vi "Add.vi"(8 "error in (no error)":errorcluster, 9 "parent tag":string, 10 "Destinations in":refnum<class "IB_Destination.lvclass">[](array[class]), 11 "userFolder in":refnum<class "userFolder.lvclass">) -> (0 "error out":errorcluster, 1 "duplicate?":bool, 2 "Destinations out":refnum<class "IB_Destination.lvclass">[](array[class]), 3 "userFolder out":refnum<class "userFolder.lvclass">)   [LabVIEW 2020, in "userFolder.lvclass"]
uses:
  <vilib>/AppBuilder/IB_Classes/Destination/userFolder/userFolder.lvclass
  <vilib>/AppBuilder/IB_Classes/Destination/userFolder/userFolder.lvclass/userFolder.ctl
  <vilib>/AppBuilder/IB_Classes/Destination/IB_Destination.lvclass
  e:/builds/penguin/labview/branches/2020/dev/dist/vi.lib/AppBuilder/IB_Classes/Destination/IB_Destination.lvclass
  e:/builds/penguin/labview/branches/2020/dev/dist/vi.lib/AppBuilder/IB_Classes/Destination/userFolder/userFolder.lvclass
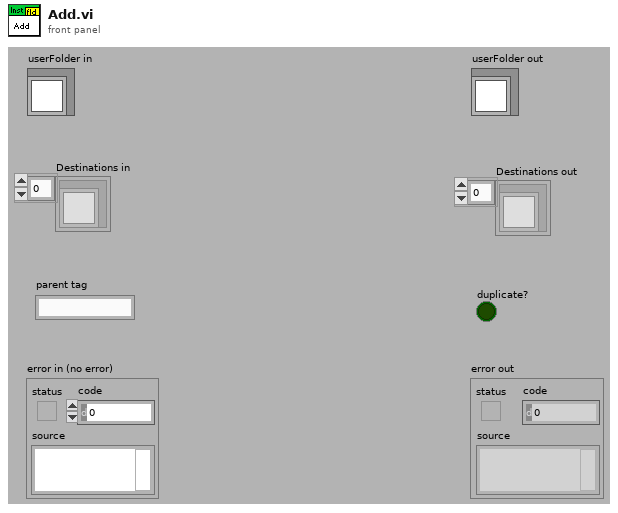
[diagram p1: front panel]
types:
  T1 = typedef "IB_Destination.ctl" = cluster{"name":string, "unlock":bool, "parentTag":string, "destTag":string, "eng_installPath":string}
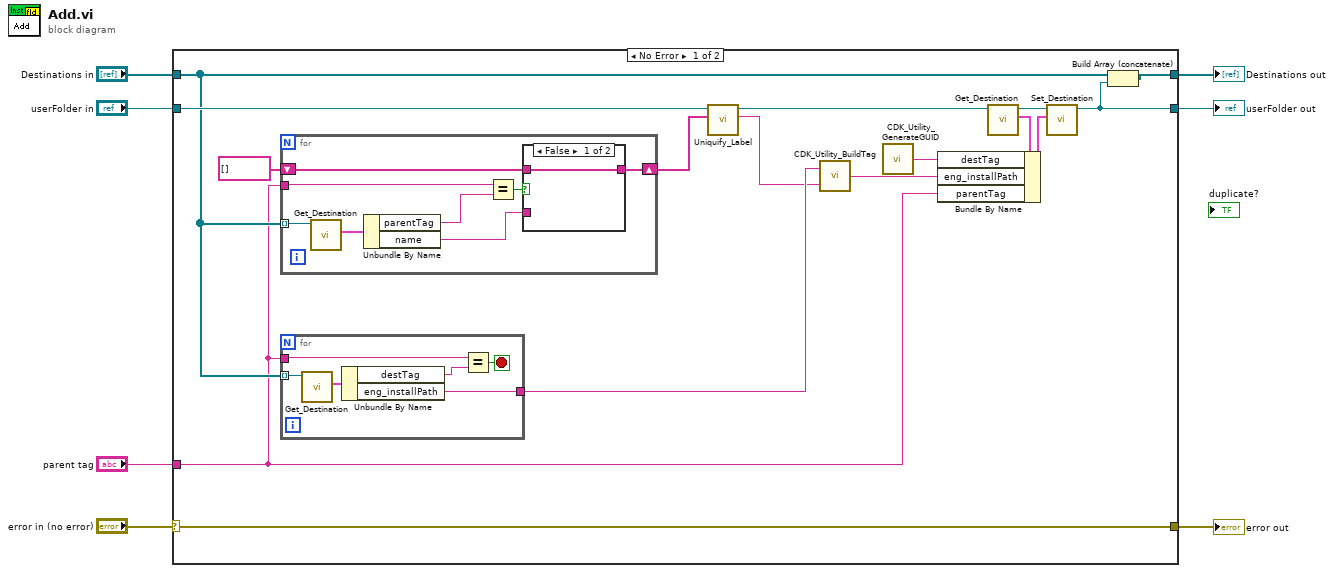
[diagram p0: block diagram]
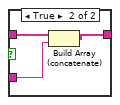
[diagram p2: hidden frame]
diagram:
  n1 = case shown="No Error" "error in (no error)" {
    selector: "error in (no error)" -> [w23 w44]
    tunnel: [w23 w44] -> w2
    tunnel: [w18 w43] -> w4
    tunnel: "userFolder in" -> [w15 w43]
    tunnel: "Destinations in" -> [w11 w42]
    tunnel: [w22 w42] -> w6
    tunnel: "parent tag" -> [w10 _]
    frame No Error {
      n2 = for {
        tunnel: w11 -> [w31] mode=indexing
        tunnel: w10 -> [w28]
        shift-right: [w25] -> w8
        shift-left: string[] [] -> [w27]
        n3 = call <vilib>:"Get_Destination.vi"("IB_Destination in"=w31) -> ("data"=w30:T1)  [unwired: 1 in, 9 out]
        n4 = Unbundle By Name(w30) -> ("parentTag"=w29:string, "name"=w24:string)
        n5 = Equal?(x=w28, y=w29) -> (x = y?=w26:bool)
        n6 = case shown="False" w26 {
          tunnel: w27 -> [w32 w35]
          tunnel: [w32 w34] -> w25
          tunnel: w24 -> [_ w33]
          frame False {
          }
          frame True {
            n7 = Build Array (concatenate)(w35, w33) -> (w34:string[])
          }
        }
      }
      n8 = for {
        tunnel: w11 -> [w41] mode=indexing
        tunnel: w10 -> [w38]
        tunnel: [w36] -> w16
        stop <- w37 stop-if-true
        n9 = call <vilib>:"Get_Destination.vi"("IB_Destination in"=w41) -> ("data"=w40:T1)  [unwired: 1 in, 9 out]
        n10 = Unbundle By Name(w40) -> ("destTag"=w39:string, "eng_installPath"=w36:string)
        n11 = Equal?(x=w38, y=w39) -> (x = y?=w37:bool)
      }
      n12 = call-dynamic "Uniquify_Label.vi"("names"=w8, "userFolder in"=w15) -> ("name"=w13:string, "userFolder out"=w14:refnum<class "userFolder.lvclass">)  [unwired: 1 in, 7 out]
      n13 = call <resource>:"CDK_Utility_BuildTag.vi"("name or relative path"=w13, "BasePath"=w16) -> ("appended path"=w17:string)
      n14 = call <resource>:"CDK_Utility_GenerateGUID.vi"() -> ("GUID"=w12:string)  [unwired: 9 out]
      n15 = call <vilib>:"Get_Destination.vi"("IB_Destination in"=w14) -> ("data"=w20:T1, "IB_Destination out"=w19:refnum<class "userFolder.lvclass">)  [unwired: 1 in, 8 out]
      n16 = Bundle By Name(cluster=w20, "destTag"=w12, "eng_installPath"=w17, "parentTag"=w10) -> (w21:T1)
      n17 = call <vilib>:"Set_Destination.vi"("data"=w21, "IB_Destination in"=w19) -> ("IB_Destination out"=w18:refnum<class "userFolder.lvclass">)  [unwired: 1 in, 8 out]
      n18 = Build Array (concatenate)(w11, w18) -> (w22:refnum<class "IB_Destination.lvclass">[])
    }
    frame Error {
    }
  }
  "error out" <- w2
  "userFolder out" <- w4
  "Destinations out" <- w6
